vi "Write Data Ref.vi"(8 "error in (no error)":errorcluster, 10 "Data*":refnum<vi>, 11 "Initialize in":refnum<class "Initialize.lvclass">) -> (0 "error out":errorcluster, 3 "Initialize out":refnum<class "Initialize.lvclass">)   [LabVIEW 2020, in "Initialize.lvclass"]
uses:
  Initialize.lvclass
  Initialize.lvclass/Initialize.ctl
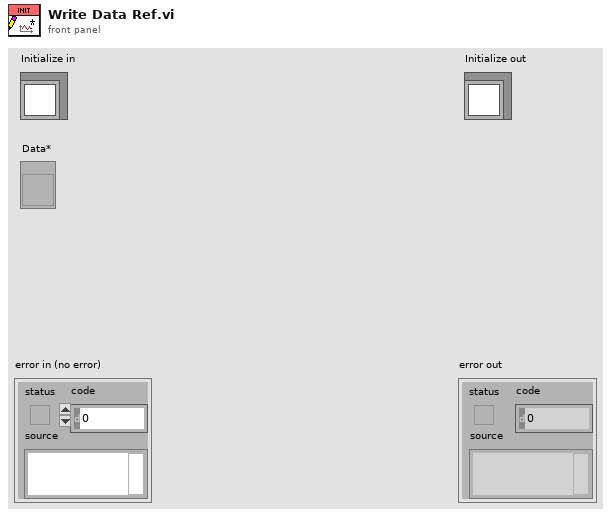
[diagram p1: front panel]
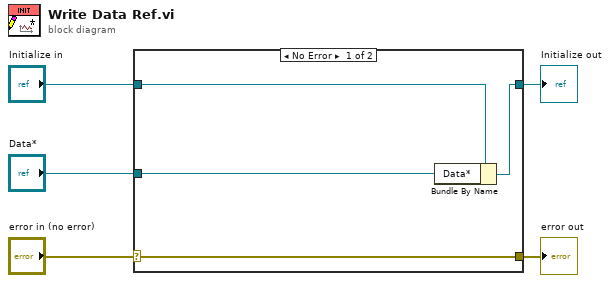
[diagram p0: block diagram]
diagram:
  n1 = case shown="No Error" "error in (no error)" {
    selector: "error in (no error)" -> [w9 w10]
    tunnel: [w9 w10] -> w4
    tunnel: [w7 w11] -> w2
    tunnel: "Initialize in" -> [w8 w11]
    tunnel: "Data*" -> [w6 _]
    frame No Error {
      n2 = Bundle By Name(cluster=w8, "Data*"=w6) -> (w7:refnum<class "Initialize.lvclass">)
    }
    frame Error {
    }
  }
  "error out" <- w4
  "Initialize out" <- w2
